vi "DoProcess.vi"(8 "error in (no error)":errorcluster, 9 "MsgQ":refnum<queue>, 10 "AbstractionActor.lvclass":refnum<class "AbstractionActor.lvclass">, 11 "ActionA in":refnum<class "ActionA.lvclass">) -> (0 "error out":errorcluster, 2 "AbstractionActor.lvclass 2":refnum<class "AbstractionActor.lvclass">, 3 "ActionA out":refnum<class "ActionA.lvclass">)   [LabVIEW 2014, in "ActionA.lvclass"]
uses:
  ActionA.lvclass
  RealWorkActor/RealWorkActor.lvclass
  AbstractionActor/AbstractionActor.lvclass
  AbstractionMessage/AbstractionMessage.lvclass
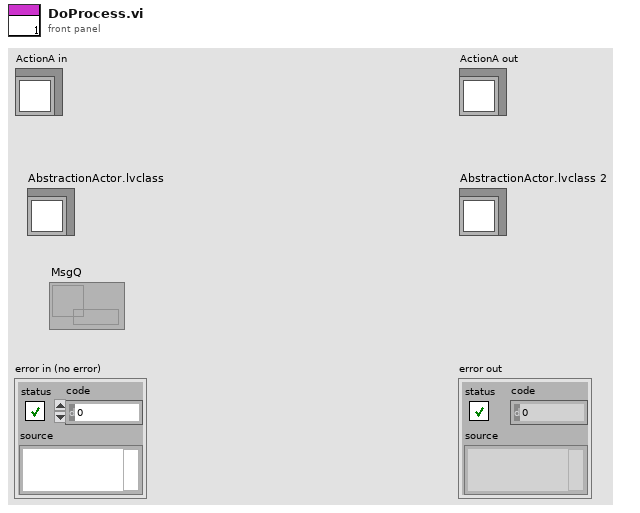
[diagram p1: front panel]
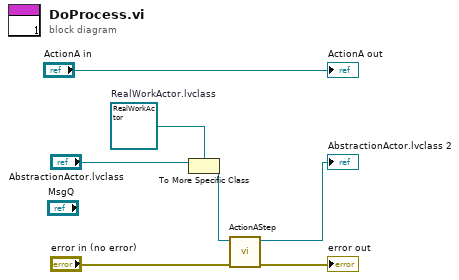
[diagram p0: block diagram]
diagram:
  w2 = refnum<class "RealWorkActor.lvclass"> refnum  # RealWorkActor.lvclass
  n1 = To More Specific Class(target class=w2, reference="AbstractionActor.lvclass") -> (specific class reference=w3:refnum<class "RealWorkActor.lvclass">)  [unwired: 1 in, 1 out]
  n2 = call "ActionAStep.vi"("error in (no error)"="error in (no error)", "RealWorkActor in"=w3) -> ("error out"=→"error out":errorcluster, "RealWorkActor out"=→"AbstractionActor.lvclass 2":refnum<class "RealWorkActor.lvclass">)  [unwired: 8 in]
  "ActionA out" <- "ActionA in"
